vi "DS345 tw sonication soft.vi"(0 "SRS DS345 GPIB address":string="0:18", 2 "Default setting (DS345)":T1={"Osc. Amp. (V)"=0.01, "Osc. Freq. (Hz)"=1000.0} {"Osc. Freq. (Hz)" min=0.001 max=250000.0 step=0.001 format="%.3f"; "Osc. Amp. (V)" min=0.0 max=0.1 step=0.001 format="%.3f"}, 3 "Cluster":T1={"Osc. Amp. (V)"=0.06, "Osc. Freq. (Hz)"=1200.0} {"Osc. Freq. (Hz)" min=1000.0 max=25000000.0 step=0.001 format="%.3f"; "Osc. Amp. (V)" min=0.01 max=10.0 step=0.01 format="%.3f"}, 4 "Lasting time (s)":dbl=10.0, 5 "Apply force":bool) -> ()   [LabVIEW 2015]
panel:
  out "Voltage (V)":dbl
  in  "Voltage velocity (V/s)":dbl=0.01 min=0.01
  out "Status (s)":dbl
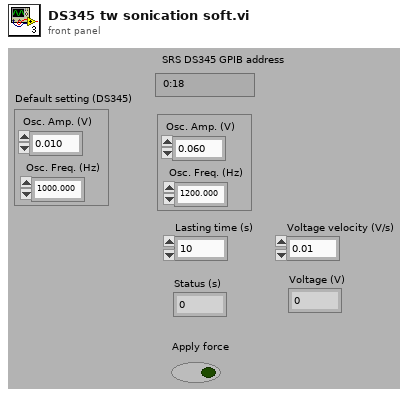
[diagram p1: front panel]
types:
  T1 = cluster{"Osc. Amp. (V)":dbl, "Osc. Freq. (Hz)":dbl}
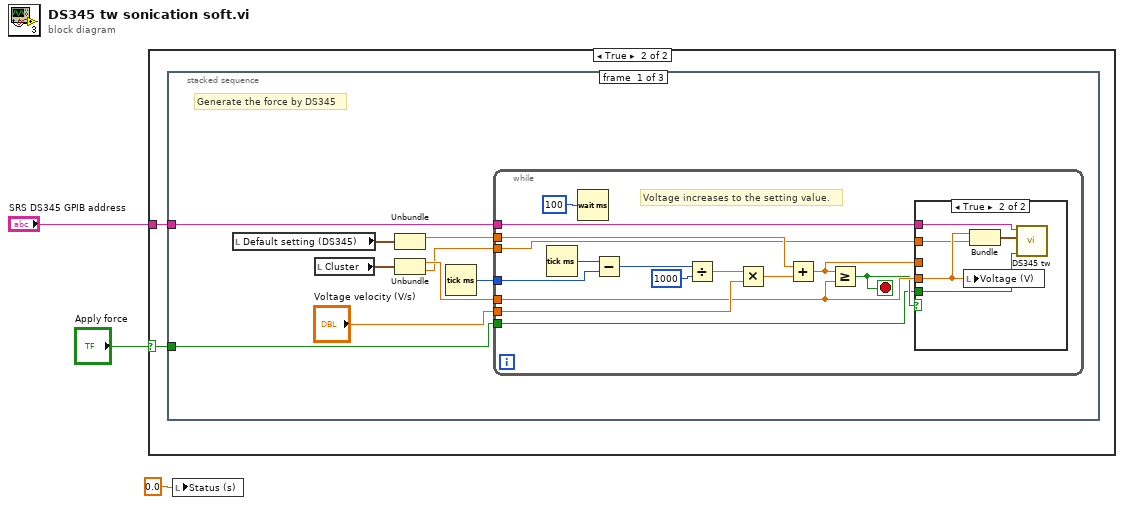
[diagram p0: block diagram]
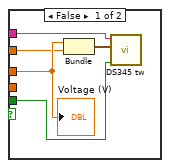
[diagram p3: hidden frame]
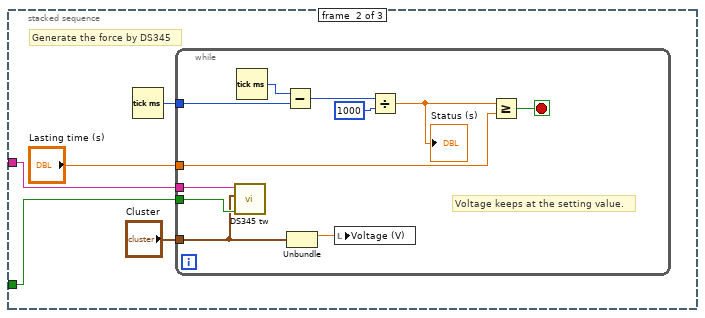
[diagram p4: hidden frame]
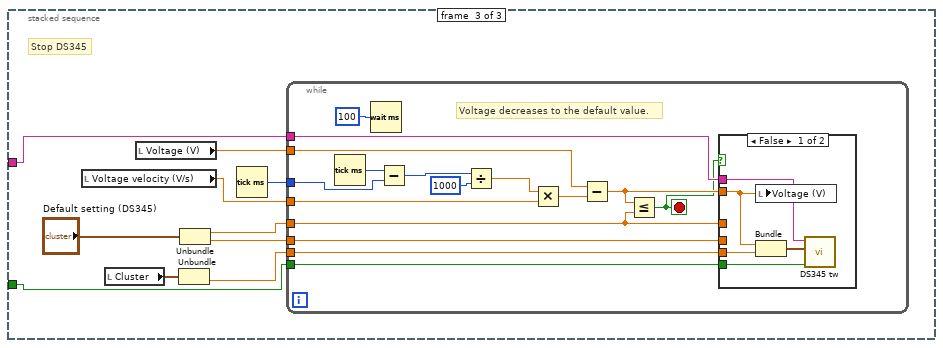
[diagram p5: hidden frame]
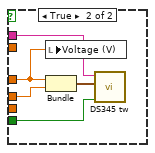
[diagram p6: hidden frame]
diagram:
  n1 = case shown="True" "Apply force" {
    selector: "Apply force" -> [_ w5]
    tunnel: "SRS DS345 GPIB address" -> [_ w4]
    frame False {
    }
    frame True {
      n2 = stacked-sequence {
        tunnel: w5 -> [w6 w41 w63]
        tunnel: w4 -> [w8 w42 w56]
        frame #0 {
          # "Generate the force by DS345"
          n3 = local read "Default setting (DS345)"() -> (w11:T1)
          n4 = local read "Cluster"() -> (w10:T1)
          n5 = Unbundle(w11) -> ("Osc. Amp. (V)"=w13:dbl)  [unwired: 1 out]
          n6 = Unbundle(w10) -> ("Osc. Amp. (V)"=w9:dbl, "Osc. Freq. (Hz)"=w7:dbl)
          n7 = Tick Count (ms)() -> (millisecond timer value=w14:u32)
          n8 = while {
            tunnel: w14 -> [w28]
            tunnel: w13 -> [w26]
            tunnel: "Voltage velocity (V/s)" -> [w22]
            tunnel: w9 -> [w20]
            tunnel: w8 -> [w17]
            tunnel: w7 -> [w16]
            tunnel: w6 -> [w15]
            stop <- w19 stop-if-true
            # "Voltage increases to the setting value."
            n9 = Tick Count (ms)() -> (millisecond timer value=w27:u32)
            n10 = Wait (ms)(milliseconds to wait=u32 100) -> ()  [unwired: 1 out]
            n11 = Subtract(x=w27, y=w28) -> (x-y=w25:u32)
            n12 = Divide(x=w25, y=u32 1000) -> (x/y=w23:dbl)
            n13 = Multiply(x=w23, y=w22) -> (x*y=w21:dbl)
            n14 = Add(x=w26, y=w21) -> (x+y=w18:dbl)
            n15 = Greater Or Equal?(x=w18, y=w20) -> (x >= y?=w19:bool)
            n16 = case shown="True" w19 {
              tunnel: w20 -> [_ w39]
              tunnel: w18 -> [w33 _]
              tunnel: w17 -> [w34 w35]
              tunnel: w16 -> [w32 w38]
              tunnel: w15 -> [w30 w36]
              frame False {
                n17 = Bundle(w33, "Osc. Freq. (Hz)"=w32) -> (w31:cluster{dbl, "Osc. Freq. (Hz)":dbl})  [unwired: 1 in]
                n18 = call "DS345 tw.vi"("Update"=w30, "Cluster"=w31, "SRS DS345 GPIB address"=w34) -> ()  [unwired: 9 in]
                "Voltage (V)" <- w33
              }
              frame True {
                n19 = local write "Voltage (V)"(w39) -> ()
                n20 = Bundle("Osc. Amp. (V)"=w39, "Osc. Freq. (Hz)"=w38) -> (w37:T1)  [unwired: 1 in]
                n21 = call "DS345 tw.vi"("Update"=w36, "Cluster"=w37, "SRS DS345 GPIB address"=w35) -> ()  [unwired: 9 in]
              }
            }
          }
        }
        frame #1 {
          # "Generate the force by DS345"
          n22 = Tick Count (ms)() -> (millisecond timer value=w44:u32)
          n23 = while {
            tunnel: w44 -> [w54]
            tunnel: "Lasting time (s)" -> [w50]
            tunnel: w42 -> [w48]
            tunnel: w41 -> [w47]
            tunnel: "Cluster" -> [w46]
            stop <- w53 stop-if-true
            # "Voltage keeps at the setting value."
            n24 = call "DS345 tw.vi"("Update"=w47, "Cluster"=w46, "SRS DS345 GPIB address"=w48) -> ()  [unwired: 9 in]
            n25 = Tick Count (ms)() -> (millisecond timer value=w55:u32)
            n26 = Subtract(x=w55, y=w54) -> (x-y=w52:u32)
            n27 = Unbundle(w46) -> ("Osc. Amp. (V)"=w45:dbl)  [unwired: 1 out]
            n28 = local write "Voltage (V)"(w45) -> ()
            n29 = Divide(x=w52, y=u32 1000) -> (x/y=w49:dbl)
            "Status (s)" <- w49
            n30 = Greater Or Equal?(x=w49, y=w50) -> (x >= y?=w53:bool)
          }
        }
        frame #2 {
          # "Stop DS345"
          n31 = local read "Voltage velocity (V/s)"() -> (w64:dbl)
          n32 = local read "Cluster"() -> (w58:T1)
          n33 = local read "Voltage (V)"() -> (w62:dbl)
          n34 = Unbundle(w58) -> ("Osc. Freq. (Hz)"=w57:dbl)  [unwired: 1 out]
          n35 = Unbundle("Default setting (DS345)") -> ("Osc. Amp. (V)"=w60:dbl, "Osc. Freq. (Hz)"=w59:dbl)
          n36 = Tick Count (ms)() -> (millisecond timer value=w65:u32)
          n37 = while {
            tunnel: w65 -> [w80]
            tunnel: w62 -> [w78]
            tunnel: w64 -> [w74]
            tunnel: w60 -> [w72]
            tunnel: w56 -> [w70]
            tunnel: w63 -> [w69]
            tunnel: w59 -> [w67]
            tunnel: w57 -> [w66]
            stop <- w68 stop-if-true
            # "Voltage decreases to the default value."
            n38 = Tick Count (ms)() -> (millisecond timer value=w79:u32)
            n39 = Wait (ms)(milliseconds to wait=u32 100) -> ()  [unwired: 1 out]
            n40 = Subtract(x=w79, y=w80) -> (x-y=w77:u32)
            n41 = Divide(x=w77, y=u32 1000) -> (x/y=w75:dbl)
            n42 = Multiply(x=w75, y=w74) -> (x*y=w73:dbl)
            n43 = Subtract(x=w78, y=w73) -> (x-y=w71:dbl)
            n44 = Less Or Equal?(x=w71, y=w72) -> (x <= y?=w68:bool)
            n45 = case shown="False" w68 {
              tunnel: w72 -> [_ w87]
              tunnel: w71 -> [w83 _]
              tunnel: w70 -> [w86 w91]
              tunnel: w69 -> [w85 w90]
              tunnel: w67 -> [_ w89]
              tunnel: w66 -> [w82 _]
              frame False {
                n46 = local write "Voltage (V)"(w83) -> ()
                n47 = Bundle(w83, "Osc. Freq. (Hz)"=w82) -> (w84:cluster{dbl, "Osc. Freq. (Hz)":dbl})  [unwired: 1 in]
                n48 = call "DS345 tw.vi"("Update"=w85, "Cluster"=w84, "SRS DS345 GPIB address"=w86) -> ()  [unwired: 9 in]
              }
              frame True {
                n49 = local write "Voltage (V)"(w87) -> ()
                n50 = Bundle("Osc. Amp. (V)"=w87, "Osc. Freq. (Hz)"=w89) -> (w88:T1)  [unwired: 1 in]
                n51 = call "DS345 tw.vi"("Update"=w90, "Cluster"=w88, "SRS DS345 GPIB address"=w91) -> ()  [unwired: 9 in]
              }
            }
          }
        }
      }
    }
  }
  n52 = local write "Status (s)"(0.0 ("Status (s)")) -> ()
